vi "Read Fault Register.vi"(8 "error in (no error)":errorcluster, 9 "channel (1)":u8=1 min=1 max=4 step=1, 11 "VISA resource name":refnum<visa-resource-name>) -> (0 "error out":errorcluster, 1 "fault register":i32, 3 "VISA resource name out":refnum<visa-resource-name>)   [LabVIEW 2020, in "Agilent 6XXX Series.lvlib"]
doc: "This function reads the fault register."
uses:
  <instrlib>/Agilent 6XXX Series/Agilent 6XXX Series.lvlib
panel:
  # "*662xA only"
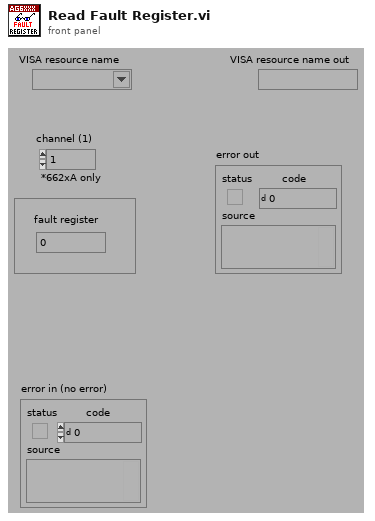
[diagram p1: front panel]
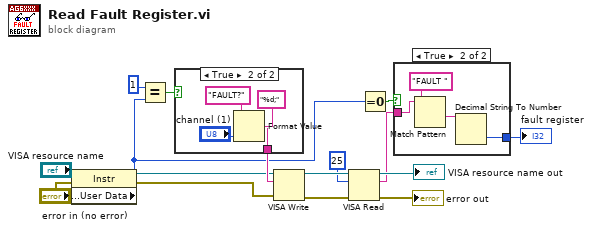
[diagram p0: block diagram]
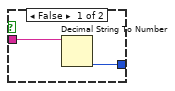
[diagram p2: hidden frame]
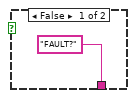
[diagram p3: hidden frame]
diagram:
  n1 = property class="Instr"(reference="VISA resource name", error in="error in (no error)") -> (reference out=w4:refnum<visa-resource-name>, error out=w3:errorcluster, "General Settings:User Data"=w5:u32)
  n2 = Equal?(x=u32 1, y=w5) -> (x = y?=w10:bool)
  n3 = case shown="True" w10 {
    tunnel: ["FAULT?" w19] -> w9
    frame False {
    }
    frame True {
      n4 = Format Value(string ("")="FAULT?", format string="%d;", value (0)="channel (1)") -> (output string=w19:string)
    }
  }
  n5 = VISA Write(VISA resource name=w4, write buffer=w9, error in (no error)=w3) -> (VISA resource name out=w16:refnum<visa-resource-name>, error out=w15:errorcluster)  [unwired: 1 out]
  n6 = VISA Read(VISA resource name=w16, byte count=u32 25, error in (no error)=w15) -> (VISA resource name out=→"VISA resource name out":refnum<visa-resource-name>, read buffer=w8:string, error out=→"error out":errorcluster)  [unwired: 1 out]
  n7 = Equal To 0?(x=w5) -> (x = 0?=w7:bool)
  n8 = case shown="True" w7 {
    tunnel: [w22 w26] -> w6
    tunnel: w8 -> [w23 w24]
    frame False {
      n9 = Decimal String To Number(string=w23) -> (number=w22:i32)  [unwired: 2 in, 1 out]
    }
    frame True {
      n10 = Match Pattern(string=w24, regular expression="FAULT ") -> (after substring=w27:string)  [unwired: 1 in, 3 out]
      n11 = Decimal String To Number(string=w27) -> (number=w26:i32)  [unwired: 2 in, 1 out]
    }
  }
  "fault register" <- w6
